vi "setLUT_action.vi"(0 "HGF_IMAQDevice in":refnum<class "HGF_IMAQDevice.lvclass">, 1 "Tap 0 LUT (Red)":u16[](array[numeric]), 2 "Tap 1 LUT (Green)":u16[](array[numeric]), 3 "Tap 2 LUT (Blue)":u16[](array[numeric]), 4 "Tap 3 LUT":u16[](array[numeric]), 5 "error in (no error)":errorcluster) -> (14 "HGF_IMAQDevice out":refnum<class "HGF_IMAQDevice.lvclass">, 19 "error out":errorcluster)   [LabVIEW 2014, in "HGF_IMAQ.lvlib" / "HGF_IMAQDevice.lvclass"]
doc: "Downloads a custom lookup table (LUT) to an image acquisition device. This VI can download 8-bit or 16-bit LUTs for analog or digital devices. If the image acquisition device has multiple LUTs, you can input all of the LUTs into this VI. Call this VI before starting the acquisition."
uses:
  HGF_IMAQDevice.lvclass
  HGF_Auxiliary/HGF_Auxiliary.lvlib
  HGF_Auxiliary/ErrorCode.ctl
  HGF_Auxiliary/Severity.ctl
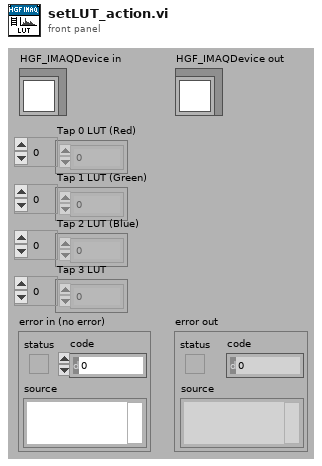
[diagram p1: front panel]
types:
  T1 = typedef "HGF_Auxiliary.lvlib/Severity.ctl" = enum16{"Info", "Warning", "Fault", "Error", "Fatal"}
  T2 = typedef "HGF_Auxiliary.lvlib/ErrorCode.ctl" = enum32{"No error", "Function not supported.", "This VI is for friends only.", "Reference object aready exisits.", "Parameter out of range.", "Not a rendezvous.", "Invalid notifier reference.", "Invalid queue reference.", "Self-Test not supported.", "Reset not supported.", "IDN query not supported.", "Error query not supported.", "Incorrect addressee.", "Object already exists.", "No class name specified", "Driver not supported", "Attribute is not writable"}
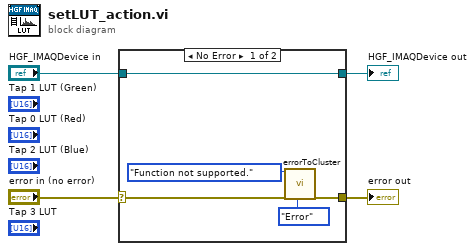
[diagram p0: block diagram]
diagram:
  n1 = case shown="No Error" "error in (no error)" {
    selector: "error in (no error)" -> [w8 w11]
    tunnel: [w5 w11] -> w3
    tunnel: [w9 w10] -> w1
    tunnel: "HGF_IMAQDevice in" -> [w9 w10]
    frame No Error {
      n2 = call "errorToCluster.vi"("error code"=ErrorCode."Function not supported.", "error in (no error)"=w8, "severity (Error)"=Severity."Error") -> ("error out"=w5:errorcluster)  [unwired: 2 in, 14 out]
    }
    frame Error {
    }
  }
  "error out" <- w3
  "HGF_IMAQDevice out" <- w1
